vi "InspectExecute.vi"(6 "Error":errorcluster, 7 "Actor":refnum<class "Actor.lvclass">, 10 "Msg":T6 {"MsgAttribs"."AbsoluteTime" format="%<%x %.3X>T"}, 11 "Actor":T1) -> (1 "Execute":bool=TRUE, 2 "Msg":T6 {"MsgAttribs"."AbsoluteTime" format="%<%x %.3X>T"}, 3 "Actor":T1, 4 "Error":errorcluster, 5 "Actor":refnum<class "Actor.lvclass">)   [LabVIEW 2020, in "_Template.lvlib" / "{{Actor}}.lvlib" / "Actor.lvclass"]
uses:
  Actor.lvclass
  jettl/jettl/Msg/Msg.lvclass
  jettl/jettl/Metadata/Metadata.lvclass
  Actor.lvclass/Actor.ctl
  jettl/jettl/Actor/Actor.lvclass
  jettl/jettl/Origin.ctl
  jettl/jettl/jettl.lvlib
  jettl/jettl/Lifecycle.ctl
  jettl/jettl/MsgExecuteType.ctl
  jettl/jettl/MsgAttribs.ctl
  jettl/jettl/Msg.ctl
  jettl/jettl/PostSetup.ctl
  jettl/jettl/PreSetup.ctl
  jettl/jettl/MsgNames.ctl
  jettl/jettl/ActorAttribs.ctl
  jettl/jettl/ChildActors.ctl
  jettl/jettl/Actor.ctl
panel:
  # "This front panel should not be manipulated."
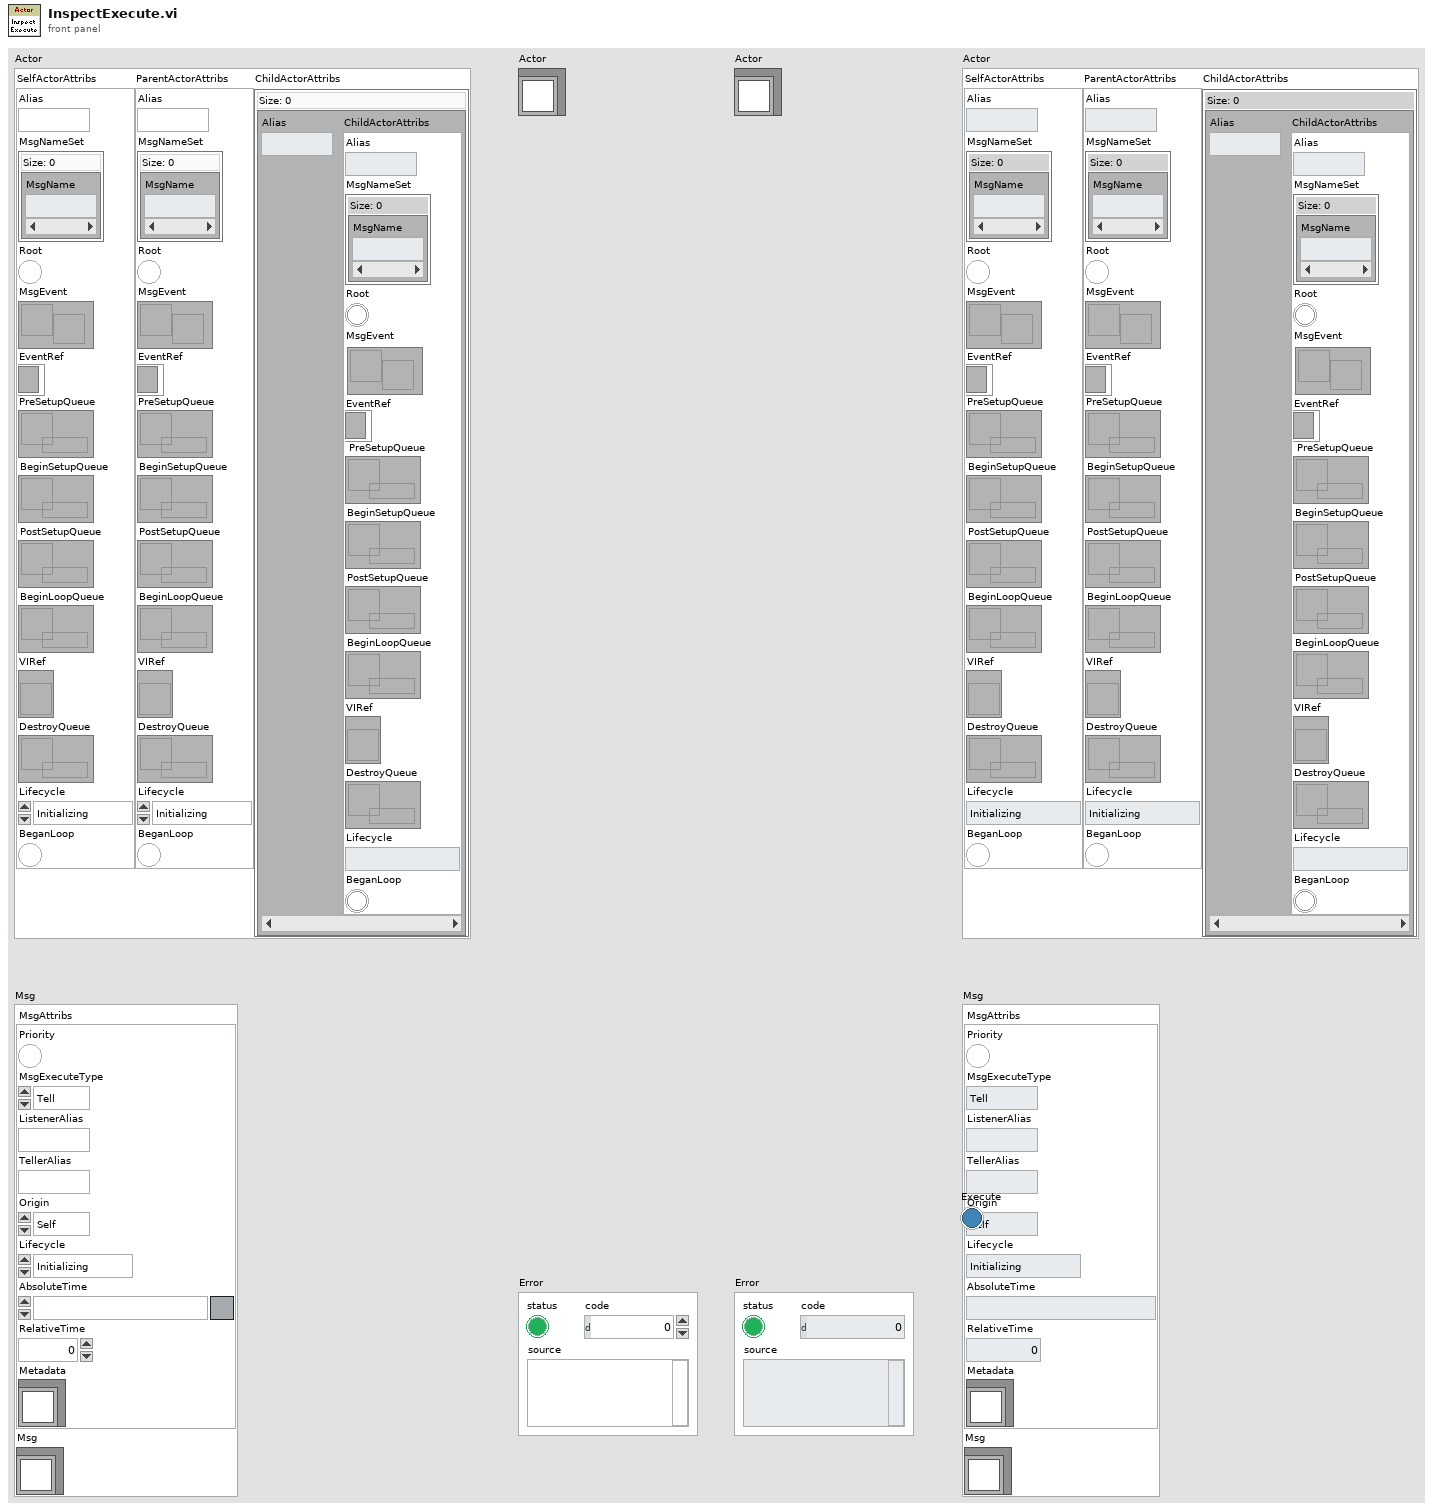
[diagram p1: front panel]
types:
  T1 = typedef "jettl.lvlib/Actor.ctl" = cluster{"SelfActorAttribs":T2, "ParentActorAttribs":T2, "ChildActorAttribs":T5}
  T2 = typedef "jettl.lvlib/ActorAttribs.ctl" = cluster{"Alias":string, "MsgNameSet":T3, "Root":bool, "MsgEvent":refnum<user-event>, "EventRef":refnum<event-registration>, "PreSetupQueue":refnum<queue>, "BeginSetupQueue":refnum<queue>, "PostSetupQueue":refnum<queue>, "BeginLoopQueue":refnum<queue>, "VIRef":refnum<vi>, "DestroyQueue":refnum<queue>, "Lifecycle":T4, "BeganLoop":bool}
  T3 = typedef "jettl.lvlib/MsgNames.ctl" = set{string}
  T4 = typedef "jettl.lvlib/Lifecycle.ctl" = enum16{"Initializing", "SettingUp", "Starting", "Running", "Stopping", "TearingDown", "Terminated"}
  T5 = typedef "jettl.lvlib/ChildActors.ctl" = map{string, T2}
  T6 = typedef "jettl.lvlib/Msg.ctl" = cluster{"MsgAttribs":T7, "Msg":refnum<class "Msg.lvclass">}
  T7 = typedef "jettl.lvlib/MsgAttribs.ctl" = cluster{"Priority":bool, "MsgExecuteType":T8, "ListenerAlias":string, "TellerAlias":string, "Origin":T9, "Lifecycle":T4, "AbsoluteTime":timestamp, "RelativeTime":dbl, "Metadata":refnum<class "Metadata.lvclass">}
  T8 = typedef "jettl.lvlib/MsgExecuteType.ctl" = enum16{"Tell", "Call"}
  T9 = typedef "jettl.lvlib/Origin.ctl" = enum16{"Self", "Parent", "Child"}
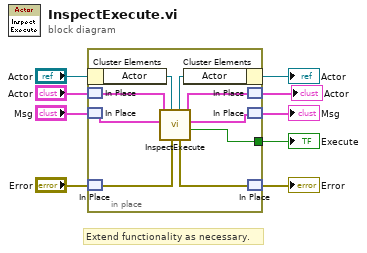
[diagram p0: block diagram]
diagram:
  # "Extend functionality as necessary."
  n1 = in-place {
    in-place-border: [w14] -> w3
    n2 = in-place-cluster #1("Actor") -> ("Actor"=w18:refnum<class "Actor.lvclass">)
    n3 = in-place-match #2("Actor") -> (w11:T1)
    n4 = in-place-match #3("Msg") -> (w12:T6)
    n5 = in-place-match #4("Error") -> (w16:errorcluster)
    n6 = call-dynamic "InspectExecute.vi"("Error"=w16, 7:"Actor"=w18, "Msg"=w12, 11:"Actor"=w11) -> ("Execute"=w14:bool, "Msg"=w13:T6, 3:"Actor"=w10:T1, "Error"=w15:errorcluster, 5:"Actor"=w17:refnum<class "Actor.lvclass">)  [unwired: 3 in]
    n7 = in-place-cluster #1("Actor"=w17) -> (→"Actor":refnum<class "Actor.lvclass">)
    n8 = in-place-match #2(w10) -> (→"Actor":T1)
    n9 = in-place-match #3(w13) -> (→"Msg":T6)
    n10 = in-place-match #4(w15) -> (→"Error":errorcluster)
  }
  "Execute" <- w3
